vi "eventmachine-bak.vi"() -> ()   [LabVIEW 2020]
panel:
  in  "EventData":T1
  out "data":i32
  in  "Stop":bool
  in  "UserEvents":T2
  out "error out":errorcluster
  in  "error in":errorcluster
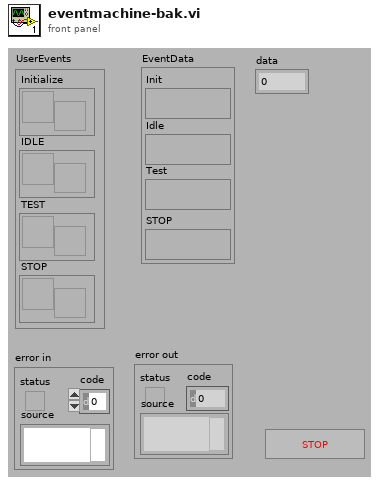
[diagram p1: front panel]
types:
  T1 = cluster{"Init":variant, "Idle":variant, "Test":variant, "STOP":variant}
  T2 = cluster{"Initialize":refnum<user-event>, "IDLE":refnum<user-event>, "TEST":refnum<user-event>, "STOP":refnum<user-event>}
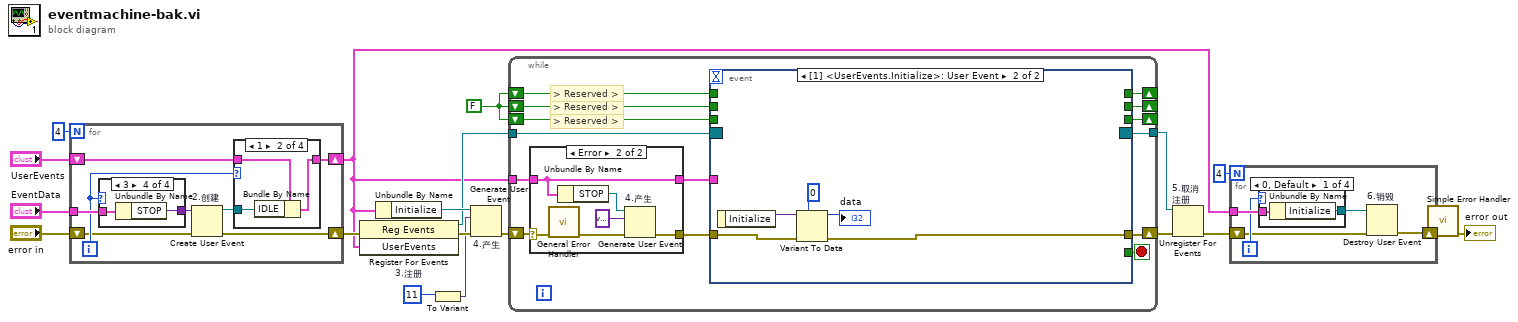
[diagram p0: block diagram]
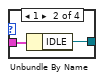
[diagram p2: hidden frame]
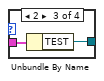
[diagram p3: hidden frame]
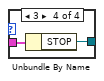
[diagram p4: hidden frame]
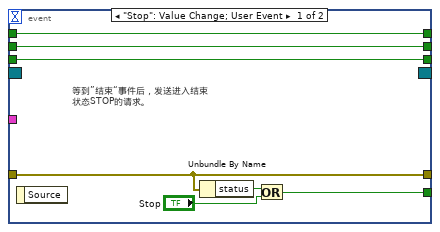
[diagram p5: hidden frame]
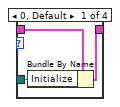
[diagram p7: hidden frame]
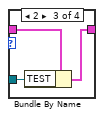
[diagram p8: hidden frame]
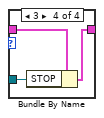
[diagram p9: hidden frame]
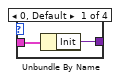
[diagram p10: hidden frame]
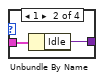
[diagram p11: hidden frame]
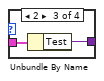
[diagram p12: hidden frame]
diagram:
  w5 = FALSE
  n1 = for {
    N: 4 -> [_]
    tunnel: "EventData" -> [w27]
    shift-right: [w22] -> w15
    shift-left: "error in" -> [w23]
    shift-right: [w20] -> w1
    shift-left: "UserEvents" -> [w21]
    i -> [w25]
    n2 = case shown="3" w25 {
      tunnel: w27 -> [w41 w43 w45 w47]
      tunnel: [w40 w42 w44 w46] -> w26
      frame 0, Default {
        n3 = Unbundle By Name(w41) -> ("Init"=w40:variant)
      }
      frame 1 {
        n4 = Unbundle By Name(w43) -> ("Idle"=w42:variant)
      }
      frame 2 {
        n5 = Unbundle By Name(w45) -> ("Test"=w44:variant)
      }
      frame 3 {
        n6 = Unbundle By Name(w47) -> ("STOP"=w46:variant)
      }
    }
    n7 = Create User Event "2.创建"(user event datatype=w26, error in=w23) -> (user event=w24:refnum<user-event>, error out=w22:errorcluster)
    n8 = case shown="1" w25 {
      tunnel: w24 -> [w29 w32 w36 w39]
      tunnel: w21 -> [w30 w33 w34 w38]
      tunnel: [w28 w31 w35 w37] -> w20
      frame 0, Default {
        n9 = Bundle By Name(cluster=w30, "Initialize"=w29) -> (w28:T2)
      }
      frame 1 {
        n10 = Bundle By Name(cluster=w33, "IDLE"=w32) -> (w31:T2)
      }
      frame 2 {
        n11 = Bundle By Name(cluster=w34, "TEST"=w36) -> (w35:T2)
      }
      frame 3 {
        n12 = Bundle By Name(cluster=w38, "STOP"=w39) -> (w37:T2)
      }
    }
  }
  n13 = register-events "3.注册"(error in=w15, w1) -> (reference out=w11:refnum<event-registration>, error out=w13:errorcluster)  [unwired: 1 in]
  n14 = Unbundle By Name(w1) -> ("Initialize"=w14:refnum<user-event>)
  n15 = To Variant(anything=11) -> (Variant=w3:variant)
  n16 = Generate User Event "4.产生"(user event=w14, event data cluster=w3, error in=w13) -> (error out=w12:errorcluster)  [unwired: 1 in, 1 out]
  n17 = while {
    shift-right: [w60] -> w9
    shift-left: w12 -> [w53]
    shift-right: [w56] -> _
    shift-left: w5 -> [w54]
    shift-right: [w59] -> _
    shift-left: w5 -> [w57]
    shift-right: [w58] -> _
    shift-left: w5 -> [w55]
    tunnel: w1 -> [w51]
    tunnel: w11 -> [w50]
    tunnel: [w49] -> w10
    stop <- w61 stop-if-true
    # "> Reserved >"
    # "> Reserved >"
    # "> Reserved >"
    n18 = case shown="Error" w53 {
      selector: w53 -> [w75 w81]
      tunnel: [w75 w79] -> w52
      tunnel: w51 -> [w74 w77]
      tunnel: [w74 w77] -> w48
      frame No Error {
      }
      frame Error {
        n19 = call <vilib>:"General Error Handler.vi"("error in (no error)"=w81) -> ("error out"=w80:errorcluster)  [unwired: 10 in, 4 out]
        n20 = Unbundle By Name(w77) -> ("STOP"=w78:refnum<user-event>)
        n21 = Generate User Event "4.产生"(user event=w78, event data cluster=variant ("event data"), error in=w80) -> (error out=w79:errorcluster)  [unwired: 1 in, 1 out]
      }
    }
    n22 = event shown="[1] <UserEvents.Initialize>: User Event" {
      selector: w50 -> [_ _]
      dyn-events: [_ _] -> w49
      timeout: _ -> [_ _]
      tunnel: w52 -> [w64 w70]
      tunnel: [w64 w69] -> w60
      tunnel: [w63 _] -> w61
      tunnel: w54 -> [w67 _]
      tunnel: w57 -> [w66 _]
      tunnel: w55 -> [w65 _]
      tunnel: [w67 _] -> w56
      tunnel: [w66 _] -> w59
      tunnel: [w65 _] -> w58
      tunnel: w48 -> [_ _]
      event "Stop": Value Change; User Event {
        # "等到”结束“事件后，发送进入结束\n状态STOP的请求。"
        n23 = event-data() -> ()  [unwired: 1 in, 1 out]
        n24 = Unbundle By Name(w64) -> ("status"=w68:bool)
        n25 = Or(x=w68, y="Stop") -> (x .or. y?=w63:bool)
      }
      event User Event {
        n26 = event-data() -> ("Initialize"=w73:variant)  [unwired: 1 in]
        n27 = Variant To Data(error in=w70, type=0, Variant=w73) -> (data=→"data":i32, error out=w69:errorcluster)
      }
    }
  }
  n28 = Unregister For Events "5.取消\n注册"(event registration refnum=w10, error in=w9) -> (error out=w7:errorcluster)
  n29 = for {
    N: 4 -> [_]
    tunnel: w1 -> [w86]
    shift-right: [w82] -> w6
    shift-left: w7 -> [w84]
    i -> [w85]
    n30 = case shown="0, Default" w85 {
      tunnel: w86 -> [w88 w90 w92 w94]
      tunnel: [w87 w89 w91 w93] -> w83
      frame 0, Default {
        n31 = Unbundle By Name(w88) -> ("Initialize"=w87:refnum<user-event>)
      }
      frame 1 {
        n32 = Unbundle By Name(w90) -> ("IDLE"=w89:refnum<user-event>)
      }
      frame 2 {
        n33 = Unbundle By Name(w92) -> ("TEST"=w91:refnum<user-event>)
      }
      frame 3 {
        n34 = Unbundle By Name(w94) -> ("STOP"=w93:refnum<user-event>)
      }
    }
    n35 = Destroy User Event "6.销毁"(user event=w83, error in=w84) -> (error out=w82:errorcluster)
  }
  n36 = call <vilib>:"Simple Error Handler.vi"("error in (no error)"=w6) -> ("error out"=→"error out":errorcluster)  [unwired: 4 in, 4 out]
